vi "Example.vi"() -> ()   [LabVIEW 2020, in "Manipulator CLI Driver.lvlib"]
uses:
  Manipulator CLI Driver.lvlib
  Manipulator Status.ctl
panel:
  in  "Move":bool
  in  "Position":dbl
  in  "Axis Index":i32
  out "Status":T1
  in  "Get Status":bool
  out "error out":errorcluster
  in  "Get Positions":bool
  out "speeds":dbl[](array[numeric])
  out "positions":dbl[](array[numeric])
  in  "stop":bool
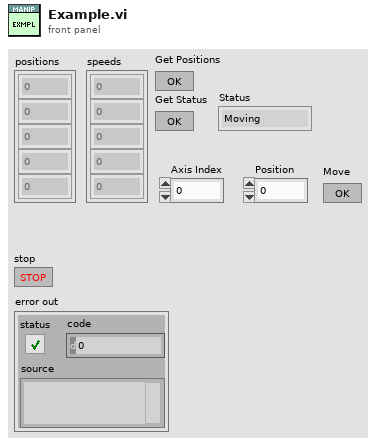
[diagram p1: front panel]
types:
  T1 = typedef "Manipulator CLI Driver.lvlib/Manipulator Status.ctl" = enum16{"Moving", "Done", "Aborted", "Error", "No Status"}
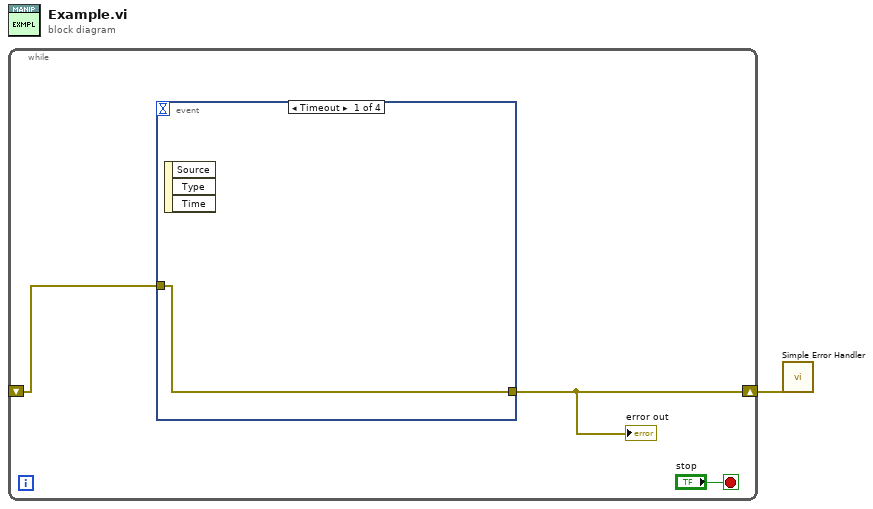
[diagram p0: block diagram]
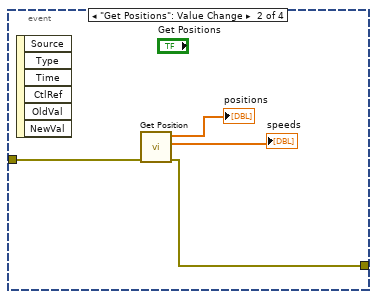
[diagram p2: hidden frame]
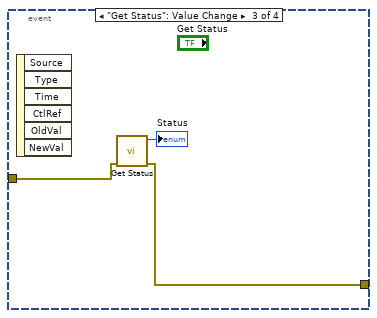
[diagram p3: hidden frame]
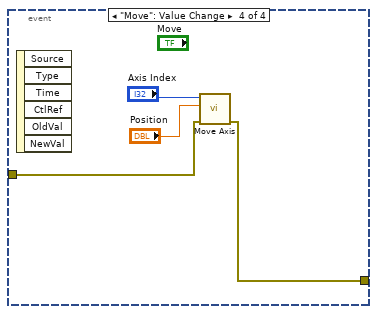
[diagram p4: hidden frame]
diagram:
  n1 = while {
    shift-right: [w3] -> w1
    shift-left: _ -> [w2]
    stop <- "stop" stop-if-true
    n2 = event shown="[0] Timeout" {
      selector: _ -> [_ _ _ _]
      dyn-events: _ -> [_ _ _ _]
      timeout: _ -> [_ _ _ _]
      tunnel: [w5 w7 w11 w13] -> w3
      tunnel: w2 -> [w5 w6 w12 w16]
      event Timeout {
        n3 = event-data() -> ()  [unwired: 1 in, 3 out]
      }
      event "Get Positions": Value Change {
        n4 = event-data() -> ()  [unwired: 1 in, 6 out]
        n5 = call "Get Position.vi"("error in (no error)"=w6) -> ("error out"=w7:errorcluster, "speeds"=→"speeds":dbl[], "positions"=→"positions":dbl[])  [unwired: 8 in]
      }
      event "Get Status": Value Change {
        n6 = event-data() -> ()  [unwired: 1 in, 6 out]
        n7 = call "Get Status.vi"("error in (no error)"=w12) -> ("error out"=w11:errorcluster, "Status"=→"Status":T1)  [unwired: 9 in]
      }
      event "Move": Value Change {
        n8 = event-data() -> ()  [unwired: 1 in, 6 out]
        n9 = call "Move Axis.vi"("error in (no error)"=w16, "Position"="Position", "Axis"="Axis Index") -> ("error out"=w13:errorcluster)  [unwired: 8 in]
      }
    }
    "error out" <- w3
  }
  n10 = call <vilib>:"Simple Error Handler.vi"("error in (no error)"=w1) -> ()  [unwired: 4 in, 5 out]
